vi "MoveCurrentToSelected.vi"(8 "error in (no error)":errorcluster, 11 "EpiWrapper in":refnum<class "EpiWrapper.lvclass">) -> (0 "error out":errorcluster, 3 "EpiWrapper out":refnum<class "EpiWrapper.lvclass">)   [LabVIEW 2012, in "EpiWrapper.lvclass"]
uses:
  EpiWrapper.lvclass
  Controls/Pad.ctl
  Controls/CurrentPad.ctl
  Controls/PadArea.ctl
  EpiWrapper.lvclass/EpiWrapper.ctl
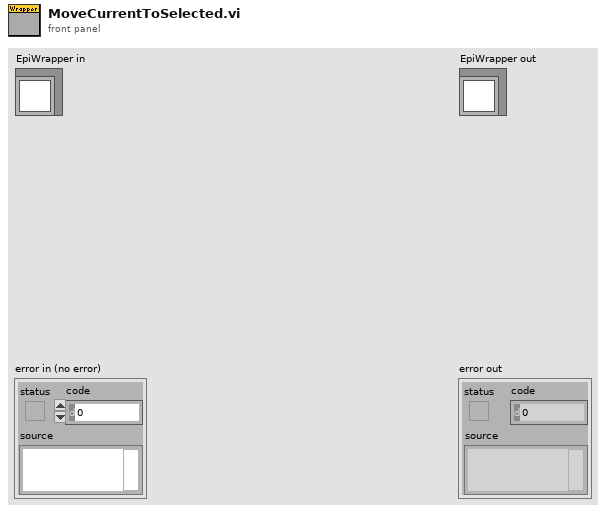
[diagram p1: front panel]
types:
  T1 = typedef "CurrentPad.ctl" = cluster{"Coords":cluster{"Horizontal":sgl, "Vertical":sgl}, "radius":i32, "Tested":bool, "Selected":bool, "Pad":string, "PadArea":T2}
  T2 = typedef "PadArea.ctl" = enum16{"A", "B", "C", "D", "L", "R", "T", "G"}
  T3 = typedef "Pad.ctl" = cluster{"Coords":cluster{"Horizontal":sgl, "Vertical":sgl}, "radius":i32, "Tested":bool, "Selected":bool, "Id":string}
  T4 = typedef "SelectedPads.ctl" = T3[]
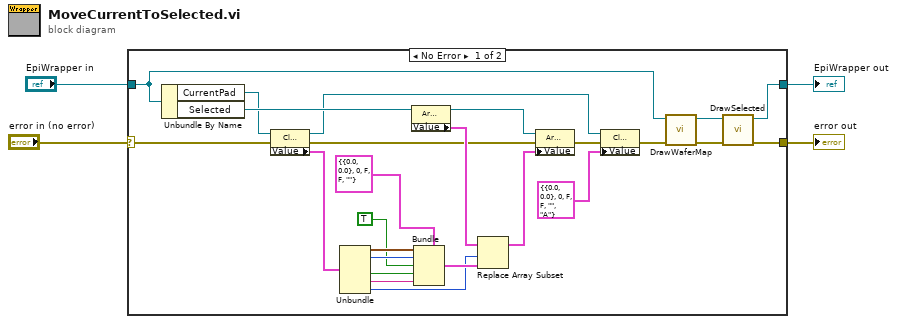
[diagram p0: block diagram]
diagram:
  n1 = case shown="No Error" "error in (no error)" {
    selector: "error in (no error)" -> [w12 w31]
    tunnel: [w11 w31] -> w3
    tunnel: [w10 w30] -> w1
    tunnel: "EpiWrapper in" -> [w6 w30]
    frame No Error {
      n2 = Unbundle By Name(w6) -> ("CurrentPad"=w25:refnum<vi>, "Selected"=w26:refnum<vi>)
      n3 = property class="Clust (strict)"(reference=w25, error in=w12) -> (reference out=w16:refnum<vi>, error out=w13:errorcluster, "Value"=w23:T1)
      n4 = Unbundle(w23) -> ("Coords"=w22:cluster{"Horizontal":sgl, "Vertical":sgl}, "radius"=w21:i32, "Selected"=w19:bool, "Pad"=w18:string, "PadArea"=w5:T2)  [unwired: 1 out]
      n5 = property class="Arr (strict)"(reference=w26) -> (reference out=w29:refnum<vi>, "Value"=w28:T4)  [unwired: 1 in, 1 out]
      n6 = Bundle(cluster=T3 {"Coords"={"Horizontal"=0.0, "Vertical"=0.0}, "radius"=0, "Tested"=FALSE, "Selected"=FALSE, "Id"=""} ("new element/subarray"), "Coords"=w22, "radius"=w21, "Tested"=TRUE, "Selected"=w19, "Id"=w18) -> (w20:T3)
      n7 = Replace Array Subset(array=w28, new element=w20, index=w5) -> (w27:T4)
      n8 = property class="Arr (strict)"(reference=w29, error in=w13, "Value"=w27) -> (error out=w14:errorcluster)  [unwired: 1 out]
      n9 = property class="Clust (strict)"(reference=w16, error in=w14, "Value"=T1 {"Coords"={"Horizontal"=0.0, "Vertical"=0.0}, "radius"=0, "Tested"=FALSE, "Selected"=FALSE, "Pad"="", "PadArea"=enum."A"}) -> (error out=w7:errorcluster)  [unwired: 1 out]
      n10 = call-dynamic "DrawWaferMap.vi"("error in (no error)"=w7, "EpiWrapper in"=w6) -> ("error out"=w8:errorcluster, "EpiWrapper out"=w9:refnum<class "EpiWrapper.lvclass">)  [unwired: 8 in]
      n11 = call-dynamic "DrawSelected.vi"("error in (no error)"=w8, "EpiWrapper in"=w9) -> ("error out"=w11:errorcluster, "EpiWrapper out"=w10:refnum<class "EpiWrapper.lvclass">)  [unwired: 8 in]
    }
    frame Error {
    }
  }
  "error out" <- w3
  "EpiWrapper out" <- w1
